vi "Write Factory Parameters.vi"(0 "Session Handle in":T1, 5 "Address":u16=171 format="%x", 7 "Bytes to Write":u8[](array[numeric]), 11 "error in (no error)":errorcluster) -> (4 "Session Handle out":T1, 15 "error out":errorcluster)   [LabVIEW 2015, in "PAS.lvclass"]
uses:
  PAS.lvclass
  Typedefs/Session Handle.ctl
panel:
  out "Whole Payload":u8[](array[numeric])
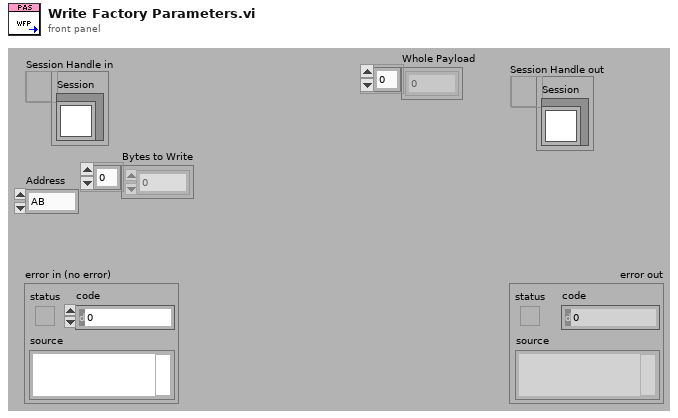
[diagram p1: front panel]
types:
  T1 = typedef "PAS.lvclass/Session Handle.ctl" = refnum<data-value>
  T2 = typedef "XNET Frame CAN.ctl" = cluster{"timestamp":timestamp, "payload":u8[], "identifier":u32, "type":T3, "extended?":bool, "echo?":bool}
  T3 = typedef "XNET Frame Type CAN.ctl" = u8
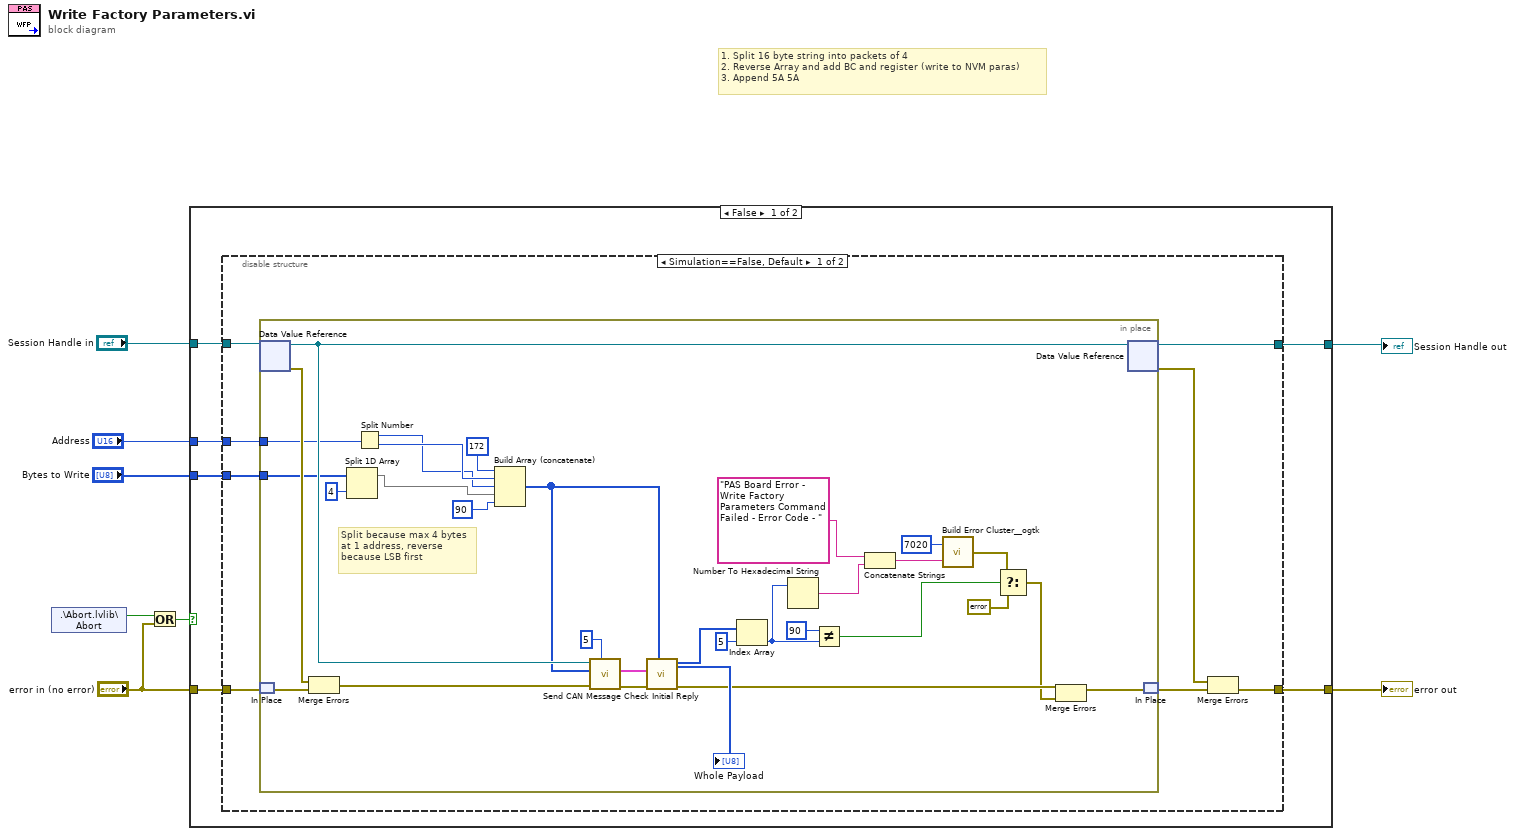
[diagram p0: block diagram]
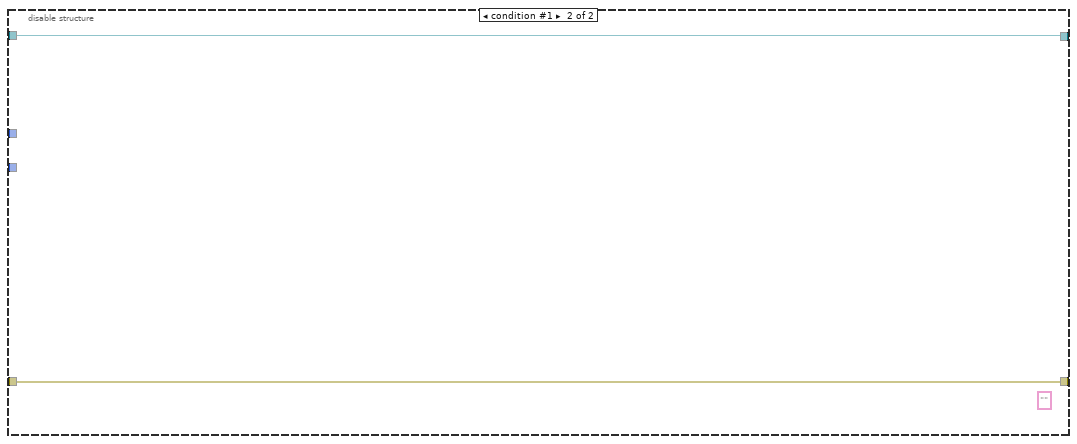
[diagram p2: hidden frame]
diagram:
  # "1. Split 16 byte string into packets of 4\n2. Reverse Array and add BC and register (write to NVM paras)\n3. Append 5A 5A"
  n1 = shared-variable ".\\Abort.lvlib\\Abort"() -> (w5:bool)  [unwired: 1 in, 1 out]
  n2 = Or(x=w5, y="error in (no error)") -> (x .or. y?=w3:bool)
  n3 = case shown="False" w3 {
    tunnel: [w14 w57] -> w7
    tunnel: [w13 w56] -> w6
    tunnel: "Session Handle in" -> [w12 w57]
    tunnel: "error in (no error)" -> [w11 w56]
    tunnel: "Address" -> [w10 _]
    tunnel: "Bytes to Write" -> [w9 _]
    frame False {
      n4 = disable-structure shown="Simulation==False, Default" {
        disable-tunnel: [w22 w55] -> w14
        disable-tunnel: [w19 w54] -> w13
        disable-tunnel: w12 -> [w18 w55]
        disable-tunnel: w11 -> [w17 w54]
        disable-tunnel: w10 -> [w16 _]
        disable-tunnel: w9 -> [w15 _]
        frame condition #0 (active) {
          n5 = in-place {
            in-place-border: w16 -> [w26]
            in-place-border: w15 -> [w32]
            # "Split because max 4 bytes\nat 1 address, reverse \nbecause LSB first"
            n6 = in-place-dvr #1(w18) -> (w50:refnum<class "PAS.lvclass">, w53:errorcluster)
            n7 = in-place-match #2(w17) -> (w52:errorcluster)
            n8 = Merge Errors(w53, w52) -> (w51:errorcluster)
            n9 = Split 1D Array(array=w32, index=4) -> (first subarray=w23:u8[])  [unwired: 1 out]
            n10 = Split Number(x=w26) -> (hi(x)=w24:u8, lo(x)=w25:u8)
            n11 = Build Array (concatenate)(u8 172, w25, w24, w23, u8 90) -> (w45:u8[])
            n12 = call "Send CAN Message.vi"("Number of Retries"=5, "error in (no error)"=w51, "payload"=w45, "Pas In"=w50) -> ("error out"=w30:errorcluster, "Reply"=w46:T2[])  [unwired: 5 in, 1 out]
            n13 = call "Check Initial Reply.vi"("Write Message"=w45, "error in (no error)"=w30, "Reply"=w46) -> ("error out"=w29:errorcluster, "Data Packet"=w41:u8[], "Whole Payload"=→"Whole Payload":u8[])  [unwired: 5 in, 1 out]
            n14 = Index Array(array=w41, index=5) -> (element=w37:u8)
            n15 = Number To Hexadecimal String(2:w37) -> (0:w36:string)  [unwired: 1 in]
            n16 = Not Equal?(x=u8 90, y=w37) -> (x != y?=w34:bool)
            n17 = Concatenate Strings("PAS Board Error - Write Factory Parameters Command Failed - Error Code - " ("string"), w36) -> (w35:string)
            n18 = call <userlib>:"Build Error Cluster__ogtk.vi"("String to Prepend to source (\"\")"=w35, "code"=7020) -> ("error out"=w43:errorcluster)
            n19 = Select(t=w43, s=w34, f=errorcluster {"status"=FALSE, "code"=0, "source"=""}) -> (s? t:f=w28:errorcluster)
            n20 = Merge Errors(w29, w28) -> (w49:errorcluster)
            n21 = in-place-dvr #1(w50) -> (w22:T1, w20:errorcluster)
            n22 = in-place-match #2(w49) -> (w21:errorcluster)
          }
          n23 = Merge Errors(w20, w21) -> (w19:errorcluster)
        }
        frame condition #1 {
          (unwired) "" ("string")
        }
      }
    }
    frame True {
    }
  }
  "Session Handle out" <- w7
  "error out" <- w6
